vi "Post to Discord.vi"(6 "Log Chat?":bool, 8 "error in (no error)":errorcluster, 10 "Mapppp":string, 11 "Image Path":path=path "C:/Users/acasalen/Desktop/testme.png") -> (0 "error out":errorcluster)   [LabVIEW 2017]
uses:
  <vilib>/httpClient/MultipartData.ctl
  <vilib>/httpClient/LabVIEWHTTPClient.lvlib
  <vilib>/Moog Components Group/Central PQS Toolkit/Miscellaneous/Miscellaneous.lvlib
panel:
  in  "Debug?":bool
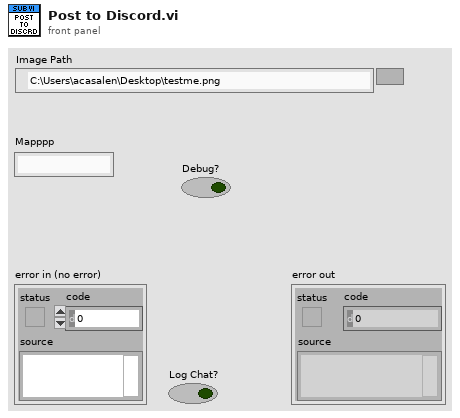
[diagram p1: front panel]
types:
  T1 = typedef "imagedata.ctl" = cluster{"image type":i32, "image depth":i32, "image":u8[], "mask":u8[], "colors":u32[], "Rectangle":cluster{"left":i16, "top":i16, "right":i16, "bottom":i16}}
  T2 = typedef "LabVIEWHTTPClient.lvlib/MultipartData.ctl" = cluster{"Name":string, "Value":string, "File":path, "Filename":string, "MIME type":string}
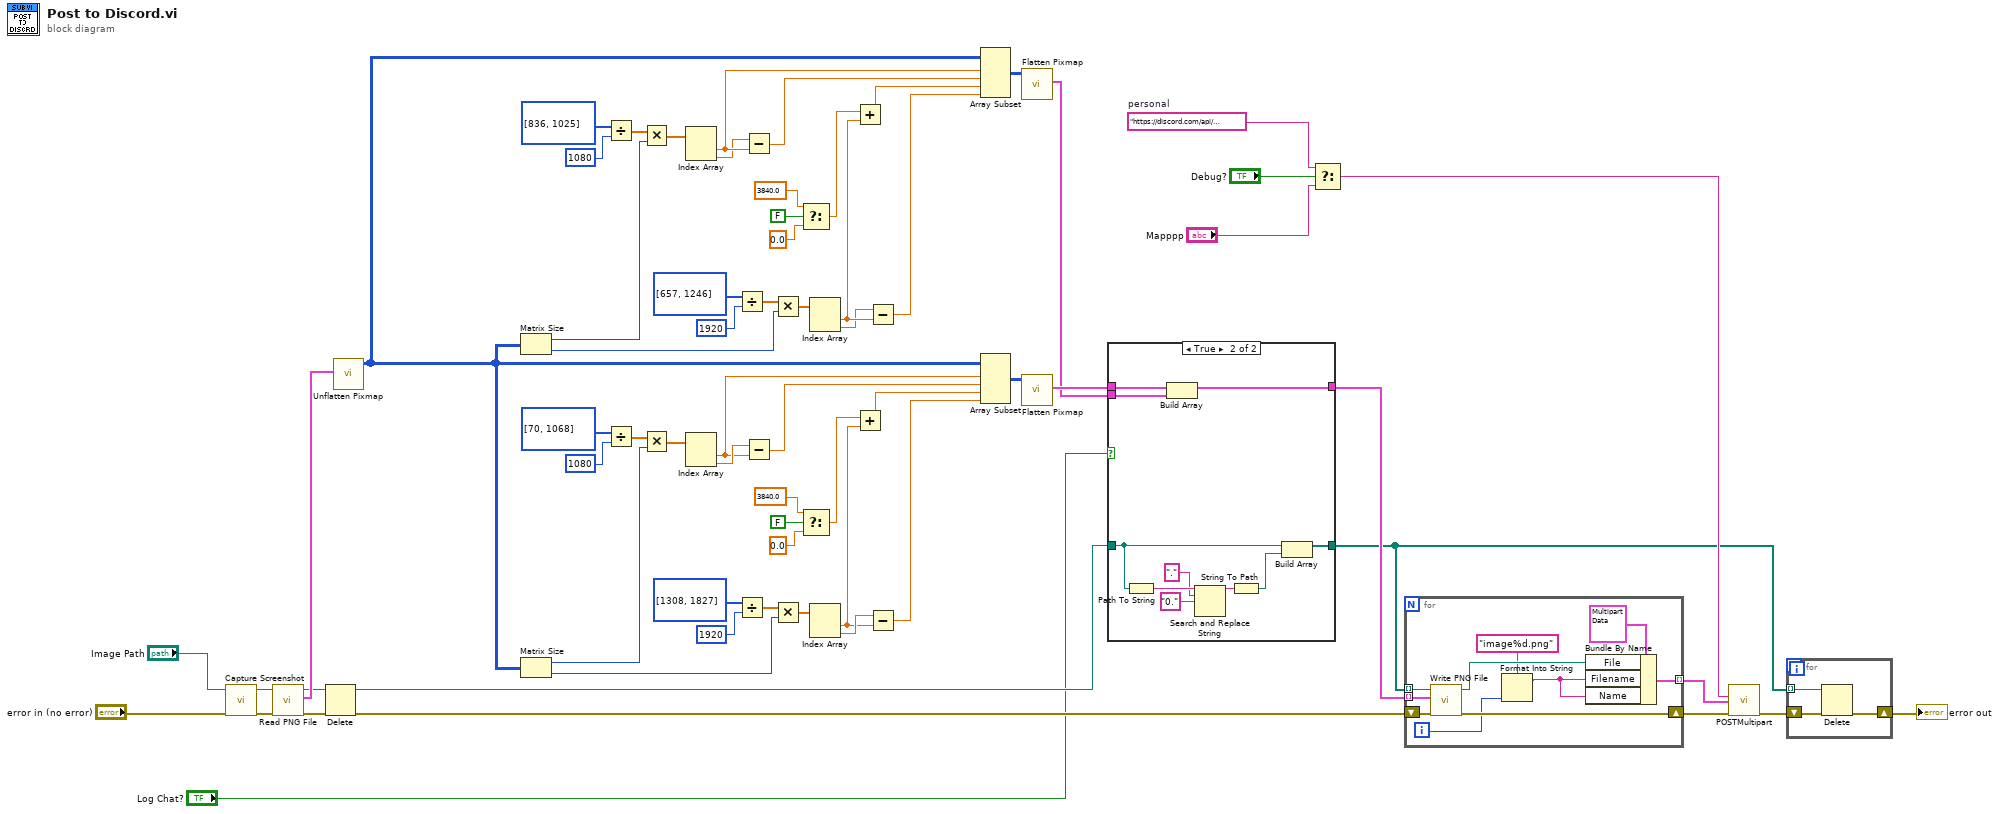
[diagram p0: block diagram]
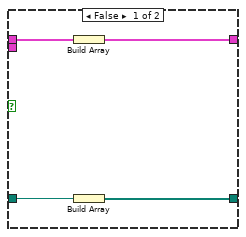
[diagram p2: hidden frame]
diagram:
  w39 = "https://discord.com/api/webhooks/888087316571242546/5E1mvxpgLwIZIkfEPfRCtBfEdzzfbidtJRk6Wlbtd9SSphCj7cs6rIf73EM-2keldoyf"  # personal
  n1 = call <vilib>:"Capture Screenshot.vi"("error in (no error)"="error in (no error)", "Image Path"="Image Path") -> ("error out"=w66:errorcluster, "dup Image Path"=w65:path)  [unwired: 8 in]
  n2 = call <vilib>:"Read PNG File.vi"("error in (no error)"=w66, "path to PNG file"=w65) -> ("error out"=w63:errorcluster, "image data"=w64:T1, "path"=w62:path)  [unwired: 7 in]
  n3 = Delete(path (use dialog)=w62, error in=w63) -> (deleted path=w14:path, error out=w47:errorcluster)  [unwired: 3 in, 1 out]
  n4 = call <vilib>:"Unflatten Pixmap.vi"("image data"=w64) -> ("24-bit pixmap"=w3:u32[][])  [unwired: 4 in, 6 out]
  n5 = Matrix Size(0:w3) -> (1:w5:i32, 2:w4:i32)
  n6 = Matrix Size(0:w3) -> (1:w1:i32, 2:w2:i32)
  n7 = Divide(x=i32[] [836, 1025], y=1080) -> (x/y=w21:dbl[])
  n8 = Divide(x=i32[] [70, 1068], y=1080) -> (x/y=w57:dbl[])
  n9 = Multiply(x=w21, y=w5) -> (x*y=w23:dbl[])
  n10 = Multiply(x=w57, y=w1) -> (x*y=w55:dbl[])
  n11 = Index Array(array=w23) -> (element #1=w25:dbl, element #2=w24:dbl)  [unwired: 2 in]
  n12 = Index Array(array=w55) -> (element #1=w53:dbl, element #2=w54:dbl)  [unwired: 2 in]
  n13 = Divide(x=i32[] [657, 1246], y=1920) -> (x/y=w22:dbl[])
  n14 = Divide(x=i32[] [1308, 1827], y=1920) -> (x/y=w56:dbl[])
  n15 = Subtract(x=w24, y=w25) -> (x-y=w26:dbl)
  n16 = Subtract(x=w54, y=w53) -> (x-y=w52:dbl)
  n17 = Multiply(x=w22, y=w4) -> (x*y=w28:dbl[])
  n18 = Multiply(x=w56, y=w2) -> (x*y=w50:dbl[])
  n19 = Select(t=3840.0 ("x"), s=FALSE, f=0.0 ("x")) -> (s? t:f=w36:dbl)
  n20 = Select(t=3840.0 ("x"), s=FALSE, f=0.0 ("x")) -> (s? t:f=w41:dbl)
  n21 = Index Array(array=w28) -> (element #1=w29:dbl, element #2=w27:dbl)  [unwired: 2 in]
  n22 = Index Array(array=w50) -> (element #1=w49:dbl, element #2=w51:dbl)  [unwired: 2 in]
  n23 = Add(x=w36, y=w29) -> (x+y=w32:dbl)
  n24 = Add(x=w41, y=w49) -> (x+y=w45:dbl)
  n25 = Subtract(x=w27, y=w29) -> (x-y=w30:dbl)
  n26 = Subtract(x=w51, y=w49) -> (x-y=w48:dbl)
  n27 = Array Subset(array=w3, index (row)=w25, length (row)=w26, index (col)=w32, length (col)=w30) -> (w31:u32[][])
  n28 = Array Subset(array=w3, index (row)=w53, length (row)=w52, index (col)=w45, length (col)=w48) -> (w46:u32[][])
  n29 = call <vilib>:"Flatten Pixmap.vi"("24-bit pixmap"=w31) -> ("image data"=w15:T1)  [unwired: 10 in]
  n30 = call <vilib>:"Flatten Pixmap.vi"("24-bit pixmap"=w46) -> ("image data"=w16:T1)  [unwired: 10 in]
  n31 = case shown="True" "Log Chat?" {
    tunnel: w16 -> [w68 w81]
    tunnel: w15 -> [_ w80]
    tunnel: w14 -> [w70 w75]
    tunnel: [w71 w76] -> w12
    tunnel: [w69 w74] -> w8
    frame False {
      n32 = Build Array(w68) -> (w71:T1[])
      n33 = Build Array(w70) -> (w69:path[])
    }
    frame True {
      n34 = Path To String(path=w75) -> (string=w79:string)
      n35 = Build Array(w81, w80) -> (w76:T1[])
      n36 = Search and Replace String(input string=w79, search string=".", replace string="0." ("replace string (\"\")")) -> (result string=w73:string)  [unwired: 5 in, 3 out]
      n37 = String To Path(string=w73) -> (path=w72:path)
      n38 = Build Array(w75, w72) -> (w74:path[])
    }
  }
  n39 = Select(t=w39, s="Debug?", f="Mapppp") -> (s? t:f=w37:string)
  n40 = for {
    shift-right: [w86] -> w10
    shift-left: w47 -> [w90]
    tunnel: w8 -> [w88] mode=indexing
    tunnel: w12 -> [w87] mode=indexing
    tunnel: [w85] -> w11 mode=indexing
    i -> [w83]
    n41 = call <vilib>:"Write PNG File.vi"("error in (no error)"=w90, "image data"=w87, "path to PNG file"=w88) -> ("error out"=w86:errorcluster, "path"=w89:path)  [unwired: 7 in]
    n42 = Format Into String(format string="image%d.png" ("Filename"), w83) -> (resulting string=w82:string)  [unwired: 2 in, 1 out]
    n43 = Bundle By Name(cluster=T2 {"Name"="", "Value"="", "File"=path "", "Filename"="", "MIME type"="application/octet-stream"} ("Element"), "File"=w89, "Filename"=w82, "Name"=w82) -> (w85:T2)
  }
  n44 = call <vilib>:"POSTMultipart.vi"("url"=w37, "data"=w11, "error in (no error)"=w10) -> ("error out"=w9:errorcluster)  [unwired: 9 in, 3 out]
  n45 = for {
    shift-right: [w93] -> w7
    shift-left: w9 -> [w94]
    tunnel: w8 -> [w92] mode=indexing
    n46 = Delete(path (use dialog)=w92, error in=w94) -> (error out=w93:errorcluster)  [unwired: 3 in, 2 out]
  }
  "error out" <- w7
